vi "Create.vi"(8 "error in (no error)":errorcluster, 10 "State Types":T1, 11 "State Factory in":refnum<class "State Factory.lvclass">) -> (0 "error out":errorcluster, 2 "State":refnum<class "State.lvclass">, 3 "State Factory out":refnum<class "State Factory.lvclass">)   [LabVIEW 2015, in "State Factory.lvclass"]
uses:
  State Factory.lvclass
  Typedefs/State Types.ctl
  State/State.lvclass
  Offline State/Offline State.lvclass
  Fault State/Fault State.lvclass
  Standby State/Standby State.lvclass
  Disabled State/Disabled State.lvclass
  Enabled State/Enabled State.lvclass
  Wait For User Input State/Wait For User Input State.lvclass
  Perform Scan State/Perform Scan State.lvclass
  Typedefs/FAMT Typedefs.lvlib
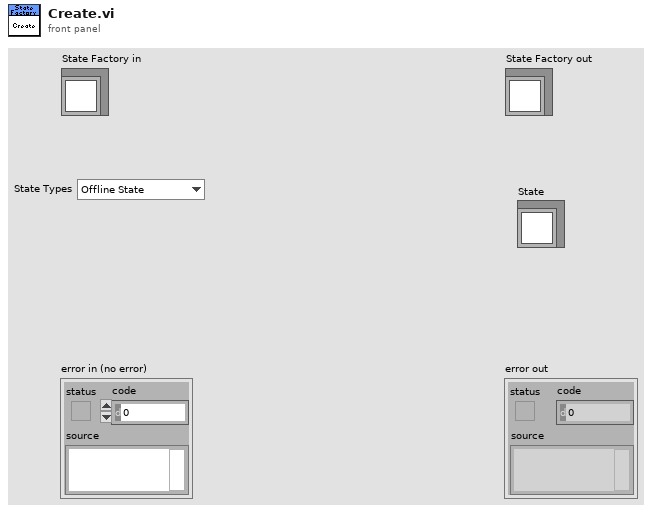
[diagram p1: front panel]
types:
  T1 = typedef "FAMT Typedefs.lvlib/State Types.ctl" = enum16{"Offline State", "Fault State", "Standby State", "Disabled State", "Enabled State", "Wait For User Input State", "Perform Scan State"}
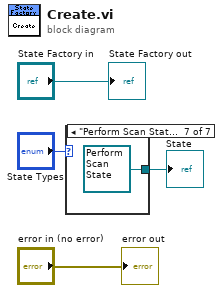
[diagram p0: block diagram]
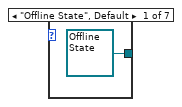
[diagram p2: hidden frame]
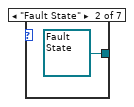
[diagram p3: hidden frame]
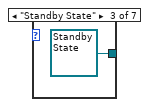
[diagram p4: hidden frame]
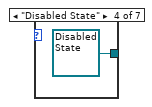
[diagram p5: hidden frame]
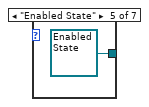
[diagram p6: hidden frame]
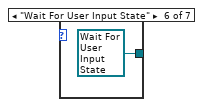
[diagram p7: hidden frame]
diagram:
  n1 = case shown="\"Perform Scan State\"" "State Types" {
    tunnel: [refnum<class "Offline State.lvclass"> refnum ("OfflineState.lvclass") refnum<class "Fault State.lvclass"> refnum ("FaultState.lvclass") refnum<class "Standby State.lvclass"> refnum ("StandbyState.lvclass") refnum<class "Disabled State.lvclass"> refnum ("DisabledState.lvclass") refnum<class "Enabled State.lvclass"> refnum ("EnabledState.lvclass") refnum<class "Wait For User Input State.lvclass"> refnum ("WaitForUserInputState.lvclass") refnum<class "Perform Scan State.lvclass"> refnum ("PerformOpenLoopScanState.lvclass")] -> w1
    frame "Offline State", Default {
    }
    frame "Fault State" {
    }
    frame "Standby State" {
    }
    frame "Disabled State" {
    }
    frame "Enabled State" {
    }
    frame "Wait For User Input State" {
    }
    frame "Perform Scan State" {
    }
  }
  "State" <- w1
  "error out" <- "error in (no error)"
  "State Factory out" <- "State Factory in"
